vi "Project File.vi"(1 "VI":refnum<vi>) -> (0 "Project File":path)   [LabVIEW 2017]
doc: "Gets the Project File (.lvproj) containg the VI."
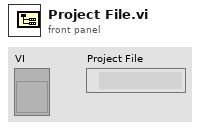
[diagram p1: front panel]
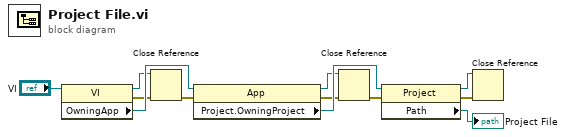
[diagram p0: block diagram]
diagram:
  n1 = property class="VI"(reference="VI") -> (reference out=w10:refnum<vi>, error out=w9:errorcluster, "OwningApp"=w12:refnum<vi>)  [unwired: 1 in]
  n2 = Close Reference(reference=w10, error in (no error)=w9) -> (error out=w8:errorcluster)
  n3 = property class="App"(reference=w12, error in=w8) -> (reference out=w7:refnum<vi>, error out=w6:errorcluster, "Project.OwningProject"=w11:refnum<vi>)
  n4 = Close Reference(reference=w7, error in (no error)=w6) -> (error out=w4:errorcluster)
  n5 = property class="Project"(reference=w11, error in=w4) -> (reference out=w5:refnum<vi>, error out=w3:errorcluster, "Path"=→"Project File":path)
  n6 = Close Reference(reference=w5, error in (no error)=w3) -> ()  [unwired: 1 out]
